vi "TESTE DE FLUXO RAFAEL.vi"() -> ()   [LabVIEW 2017]
uses:
  <vilib>/LabVIEW Interface for Arduino/Type Defs/Pin Mode.ctl
  <vilib>/LabVIEW Interface for Arduino/LabVIEW Interface for Arduino.lvlib
  <vilib>/LabVIEW Interface for Arduino/Type Defs/Board Type.ctl
  <vilib>/LabVIEW Interface for Arduino/Type Defs/Connection Type.ctl
panel:
  in  "stop":bool
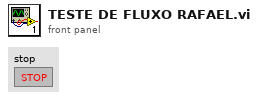
[diagram p1: front panel]
types:
  T1 = typedef "LabVIEW Interface for Arduino.lvlib/Connection Type.ctl" = enum8{"USB / Serial", "XBEE", "BlueSmirf (Bluetooth)"}
  T2 = typedef "LabVIEW Interface for Arduino.lvlib/Board Type.ctl" = enum16{"Uno", "Dimuelanove w/Atmega 328", "Mega 2560"}
  T3 = typedef "LabVIEW Interface for Arduino.lvlib/Arduino Resource.ctl" = cluster{"VISA resource":refnum<visa-resource-name>, "Board Type":T2, "Connection Type":enum8{"USB / Serial"}, "Bytes Per Packet (15)":u8}
  T4 = typedef "LabVIEW Interface for Arduino.lvlib/Pin Mode.ctl" = enum8{"Input", "Output"}
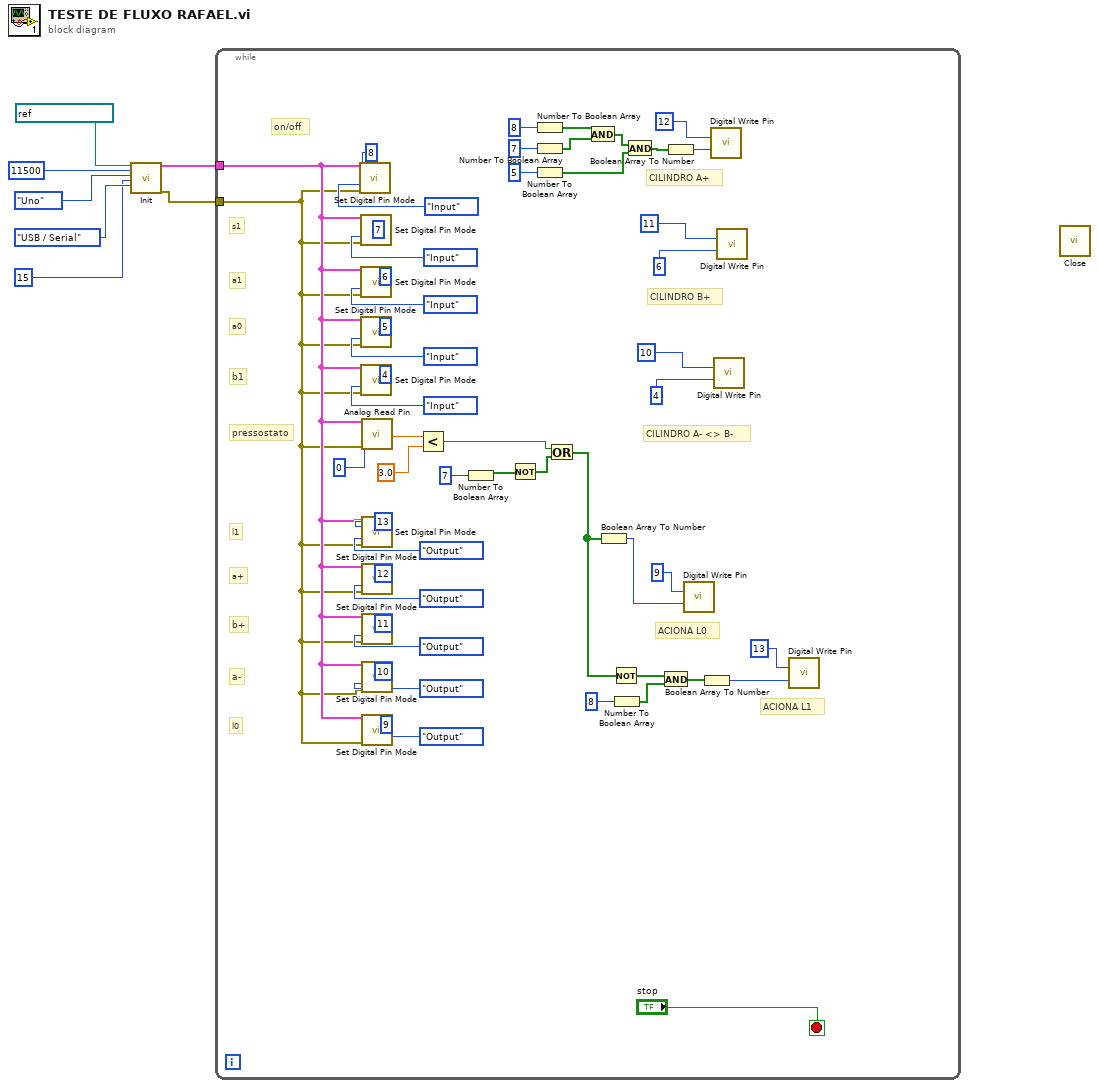
[diagram p0: block diagram]
diagram:
  n1 = call <vilib>:"Init.vi"("VISA resource"=refnum<visa-resource-name> "ASRL9::INSTR", "Baud Rate (115200)"=u32 11500, "Board Type (Uno)"=Board_Type."Uno", "Bytes Per Packet (15)"=u32 15, "Connection Type (USB/Serial)"=Connection_Type."USB / Serial") -> ("Arduino Resource"=w7:T3, "error out"=w6:errorcluster)  [unwired: 13 in]
  n2 = while {
    tunnel: w7 -> [w39]
    tunnel: w6 -> [w38]
    stop <- "stop" stop-if-true
    # "ACIONA L1"
    # "ACIONA L0"
    # "CILINDRO A- <> B-"
    # "CILINDRO B+"
    # "CILINDRO A+"
    # "l0"
    # "a-"
    # "b+"
    # "a+"
    # "l1"
    # "pressostato"
    # "b1"
    # "a0"
    # "a1"
    # "s1"
    # "on/off"
    n3 = call <vilib>:"Set Digital Pin Mode.vi"("Arduino Resource"=w39, "Digital I/O Pin"=u8 8, "Pin Mode (Input)"=Pin_Mode."Input", "error in"=w38) -> ()  [unwired: 10 in, 2 out]
    n4 = call <vilib>:"Set Digital Pin Mode.vi"("Arduino Resource"=w39, "Digital I/O Pin"=u8 7, "Pin Mode (Input)"=Pin_Mode."Input", "error in"=w38) -> ()  [unwired: 10 in, 2 out]
    n5 = call <vilib>:"Set Digital Pin Mode.vi"("Arduino Resource"=w39, "Digital I/O Pin"=u8 6, "Pin Mode (Input)"=Pin_Mode."Input", "error in"=w38) -> ()  [unwired: 10 in, 2 out]
    n6 = call <vilib>:"Set Digital Pin Mode.vi"("Arduino Resource"=w39, "Digital I/O Pin"=u8 5, "Pin Mode (Input)"=Pin_Mode."Input", "error in"=w38) -> ()  [unwired: 10 in, 2 out]
    n7 = call <vilib>:"Set Digital Pin Mode.vi"("Arduino Resource"=w39, "Digital I/O Pin"=u8 4, "Pin Mode (Input)"=Pin_Mode."Input", "error in"=w38) -> ()  [unwired: 10 in, 2 out]
    n8 = call <vilib>:"Analog Read Pin.vi"("Arduino Resource"=w39, "Analog Input Pin (0)"=u8 0, "error in"=w38) -> ("Voltage"=w20:dbl)  [unwired: 10 in, 2 out]
    n9 = call <vilib>:"Set Digital Pin Mode.vi"("Arduino Resource"=w39, "Digital I/O Pin"=u8 13, "Pin Mode (Input)"=Pin_Mode."Output", "error in"=w38) -> ()  [unwired: 10 in, 2 out]
    n10 = call <vilib>:"Set Digital Pin Mode.vi"("Arduino Resource"=w39, "Digital I/O Pin"=u8 12, "Pin Mode (Input)"=Pin_Mode."Output", "error in"=w38) -> ()  [unwired: 10 in, 2 out]
    n11 = call <vilib>:"Set Digital Pin Mode.vi"("Arduino Resource"=w39, "Digital I/O Pin"=u8 11, "Pin Mode (Input)"=Pin_Mode."Output", "error in"=w38) -> ()  [unwired: 10 in, 2 out]
    n12 = call <vilib>:"Set Digital Pin Mode.vi"("Arduino Resource"=w39, "Digital I/O Pin"=u8 10, "Pin Mode (Input)"=Pin_Mode."Output", "error in"=w38) -> ()  [unwired: 10 in, 2 out]
    n13 = call <vilib>:"Set Digital Pin Mode.vi"("Arduino Resource"=w39, "Digital I/O Pin"=u8 9, "Pin Mode (Input)"=Pin_Mode."Output", "error in"=w38) -> ()  [unwired: 10 in, 2 out]
    n14 = Less?(x=w20, y=3.0) -> (x < y?=w18:bool)
    n15 = Number To Boolean Array(number=u32 7) -> (Boolean array=w22:bool[])
    n16 = Not(x=w22) -> (.not. x?=w17:bool[])
    n17 = Number To Boolean Array(number=u32 8) -> (Boolean array=w37:bool[])
    n18 = Number To Boolean Array(number=u32 7) -> (Boolean array=w36:bool[])
    n19 = Number To Boolean Array(number=u32 5) -> (Boolean array=w31:bool[])
    n20 = Or(x=w18, y=w17) -> (x .or. y?=w14:bool[])
    n21 = And(x=w37, y=w36) -> (x .and. y?=w33:bool[])
    n22 = Boolean Array To Number(Boolean array=w14) -> (number=w16:u32)
    n23 = Not(x=w14) -> (.not. x?=w13:bool[])
    n24 = Number To Boolean Array(number=u32 8) -> (Boolean array=w12:bool[])
    n25 = And(x=w33, y=w31) -> (x .and. y?=w29:bool[])
    n26 = And(x=w13, y=w12) -> (x .and. y?=w10:bool[])
    n27 = Boolean Array To Number(Boolean array=w29) -> (number=w30:u32)
    n28 = call <vilib>:"Digital Write Pin.vi"("Digital I/O Pin (0)"=u8 9, "Value (0)"=w16) -> ()  [unwired: 12 in, 2 out]
    n29 = Boolean Array To Number(Boolean array=w10) -> (number=w8:u32)
    n30 = call <vilib>:"Digital Write Pin.vi"("Digital I/O Pin (0)"=u8 12, "Value (0)"=w30) -> ()  [unwired: 12 in, 2 out]
    n31 = call <vilib>:"Digital Write Pin.vi"("Digital I/O Pin (0)"=u8 10, "Value (0)"=u8 4) -> ()  [unwired: 12 in, 2 out]
    n32 = call <vilib>:"Digital Write Pin.vi"("Digital I/O Pin (0)"=u8 11, "Value (0)"=u8 6) -> ()  [unwired: 12 in, 2 out]
    n33 = call <vilib>:"Digital Write Pin.vi"("Digital I/O Pin (0)"=u8 13, "Value (0)"=w8) -> ()  [unwired: 12 in, 2 out]
  }
  n34 = call <vilib>:"Close.vi"() -> ()  [unwired: 15 in, 1 out]
